vi "CRYAPI Check Fit.vi"(8 "WindowNumber":i32=2, 9 "pSPRef":refnum<vi>, 10 "pPanRef":refnum<vi>) -> ()   [LabVIEW 2013]
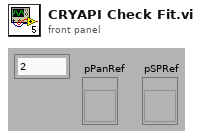
[diagram p1: front panel]
types:
  T1 = typedef "LVRectTypeDef.ctl" = cluster{"Left":i16, "Top":i16, "Right":i16, "Bottom":i16}
  T2 = cluster{"nType":i32, "nParent":i32, "pVIW":refnum<vi>, "pSPW":refnum<vi>, "nTypeF":i32, "pVIF":refnum<vi>, "pSPF":refnum<vi>, "nIDSpliter":i32, "nProperty":i32, "Bound":T1, "nID":i32, "nData":i32, "sData":string, "pWVI":refnum<vi>, "sTitle":string, "cPages":cluster{"nPage":i32, "sTitle":string, "sIcon":string, "pVI":refnum<vi>, "nID":i32}[], "pTab":refnum<vi>, "nIDPages":i32[], "pSPT":refnum<vi>, "sTemp":string, "nDockID":i32, "nDockLR":i32, "sIcon":string}
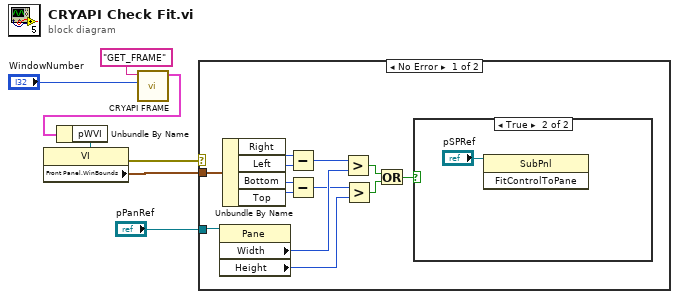
[diagram p0: block diagram]
diagram:
  n1 = call "CRYAPI FRAME.vi"("nData"="WindowNumber", "sAction"="GET_FRAME") -> ("tFrame_Out"=w6:T2)  [unwired: 4 in, 5 out]
  n2 = Unbundle By Name(w6) -> ("pWVI"=w5:refnum<vi>)
  n3 = property class="VI"(reference=w5) -> (error out=w4:errorcluster, "Front Panel.WinBounds"=w3:T1)  [unwired: 1 in, 1 out]
  n4 = case shown="No Error" w4 {
    tunnel: w3 -> [w20 _]
    tunnel: "pPanRef" -> [w19 _]
    frame No Error {
      n5 = property class="Pane"(reference=w19) -> ("Width"=w13:u32, "Height"=w11:u32)  [unwired: 1 in, 2 out]
      n6 = Unbundle By Name(w20) -> ("Right"=w17:i16, "Left"=w18:i16, "Bottom"=w15:i16, "Top"=w16:i16)
      n7 = Subtract(x=w17, y=w18) -> (x-y=w14:i16)
      n8 = Subtract(x=w15, y=w16) -> (x-y=w12:i16)
      n9 = Greater?(x=w14, y=w13) -> (0:w10:bool)
      n10 = Greater?(x=w12, y=w11) -> (0:w9:bool)
      n11 = Or(x=w10, y=w9) -> (x .or. y?=w8:bool)
      n12 = case shown="True" w8 {
        frame False {
        }
        frame True {
          n13 = invoke on="Invoke Node" class="SubPnl" method="FitControlToPane"(reference="pSPRef") -> ()  [unwired: 2 in, 3 out]
        }
      }
    }
    frame Error {
    }
  }
